vi "Uptime.vi"(11 "System Status Actor in":refnum<class "System Status Actor.lvclass">) -> (3 "System Status Actor out":refnum<class "System Status Actor.lvclass">)   [LabVIEW 2020, in "RTAF.lvlib" / "System Status Actor.lvclass"]
uses:
  System Status Actor.lvclass
  System Status Actor.lvclass/System Status Actor.ctl
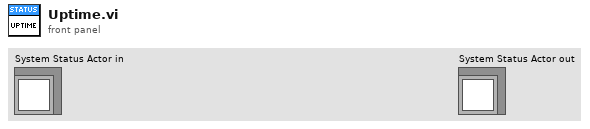
[diagram p1: front panel]
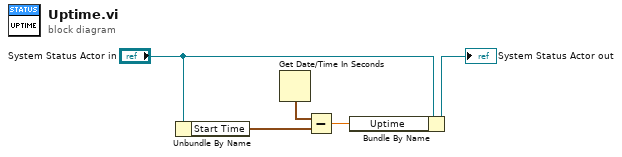
[diagram p0: block diagram]
diagram:
  n1 = Unbundle By Name("System Status Actor in") -> ("Start Time"=w2:timestamp)
  n2 = Get Date/Time In Seconds() -> (seconds since 1Jan1904=w3:timestamp)
  n3 = Subtract(x=w3, y=w2) -> (x-y=w1:dbl)
  n4 = Bundle By Name(cluster="System Status Actor in", "Uptime"=w1) -> (→"System Status Actor out":refnum<class "System Status Actor.lvclass">)
